vi "Embed Actor Core In Subpanel.vi"(8 "error in (no error)":errorcluster, 10 "Subpanel":refnum<vi>, 11 "SongBrowserActor In":refnum<class "SongBrowserActor.lvclass">) -> (0 "error out":errorcluster, 3 "SongBrowserActor Out":refnum<class "SongBrowserActor.lvclass">)   [LabVIEW 2015, in "SongBrowserActor.lvlib" / "SongBrowserActor.lvclass"]
uses:
  SongBrowserActor.lvclass
  SongBrowserActor.lvclass/SongBrowserActor.ctl
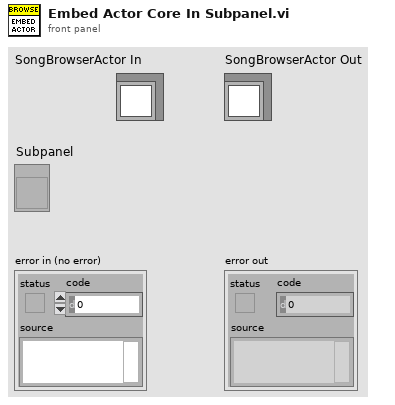
[diagram p1: front panel]
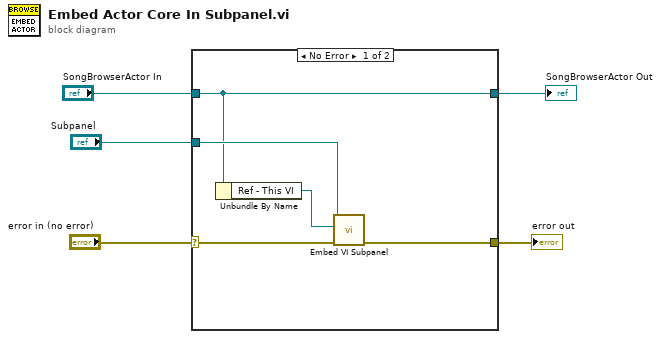
[diagram p0: block diagram]
diagram:
  n1 = case shown="No Error" "error in (no error)" {
    selector: "error in (no error)" -> [w10 w12]
    tunnel: [w9 w12] -> w4
    tunnel: [w7 w11] -> w1
    tunnel: "SongBrowserActor In" -> [w7 w11]
    tunnel: "Subpanel" -> [w8 _]
    frame No Error {
      n2 = Unbundle By Name(w7) -> ("Ref - This VI"=w6:refnum<vi>)
      n3 = call "Embed VI Subpanel.vi"("Error In"=w10, "VI Ref"=w6, "Subpanel Ref"=w8) -> ("Error Out"=w9:errorcluster)  [unwired: 8 in]
    }
    frame Error {
    }
  }
  "error out" <- w4
  "SongBrowserActor Out" <- w1
